vi "add sensors.vi"(9 "add sensors":T1(array[cluster]), 10 "sensors":T1(array[cluster])) -> (2 "sensor out":T1(array[cluster]))   [LabVIEW 2011]
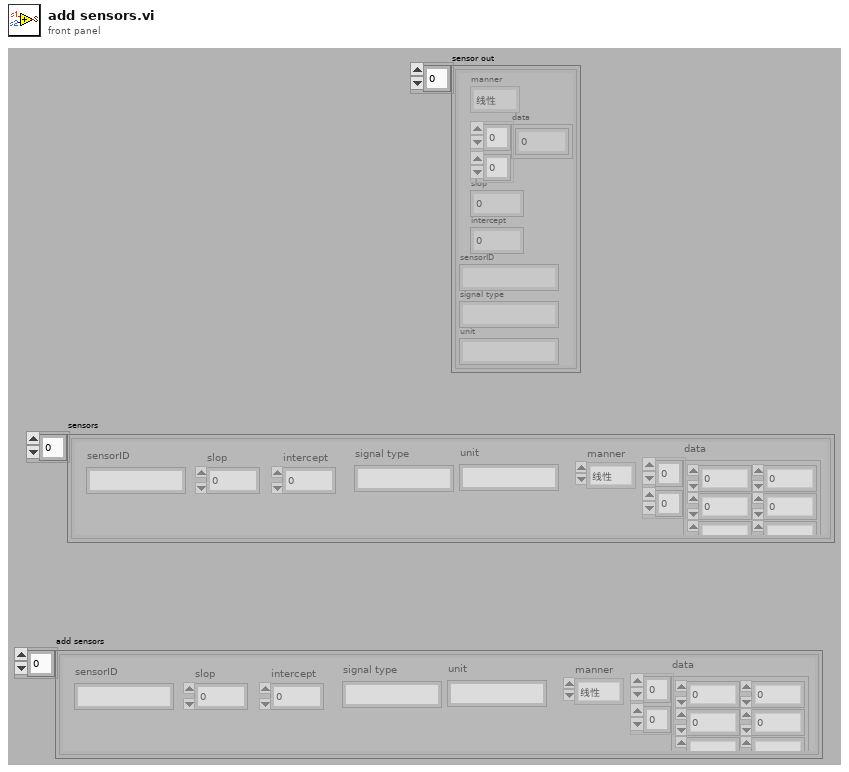
[diagram p1: front panel]
types:
  T1 = cluster{"manner":enum16{"线性", "查表"}, "data":dbl[][], "slop":dbl, "intercept":dbl, "sensorID":string, "signal type":string, "unit":string}[]
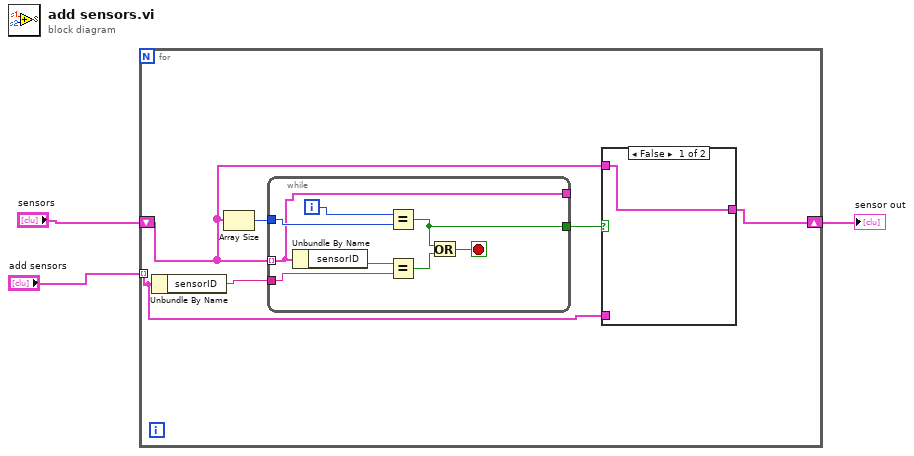
[diagram p0: block diagram]
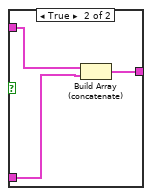
[diagram p2: hidden frame]
diagram:
  n1 = for {
    tunnel: "add sensors" -> [w6] mode=indexing
    shift-right: [w4] -> w1
    shift-left: "sensors" -> [w5]
    n2 = Unbundle By Name(w6) -> ("sensorID"=w9:string)
    n3 = Array Size(array=w5) -> (size(s)=w8:i32)
    n4 = while {
      tunnel: w5 -> [w15] mode=indexing
      tunnel: w9 -> [w20]
      tunnel: w8 -> [w19]
      tunnel: [w16] -> w7
      tunnel: [w15] -> _
      i -> [w14]
      stop <- w17 stop-if-true
      n5 = Unbundle By Name(w15) -> ("sensorID"=w21:string)
      n6 = Equal?(x=w14, y=w19) -> (x = y?=w16:bool)
      n7 = Equal?(x=w21, y=w20) -> (x = y?=w18:bool)
      n8 = Or(x=w16, y=w18) -> (x .or. y?=w17:bool)
    }
    n9 = case shown="False" w7 {
      tunnel: w6 -> [_ w12]
      tunnel: w5 -> [w10 w13]
      tunnel: [w10 w11] -> w4
      frame False {
      }
      frame True {
        n10 = Build Array (concatenate)(w13, w12) -> (w11:T1)
      }
    }
  }
  "sensor out" <- w1
